vi "ElementPositions.vi"() -> ()   [LabVIEW 2012]
panel:
  in  "Threshold":dbl
  in  "ElementPositions":T1(array[cluster])
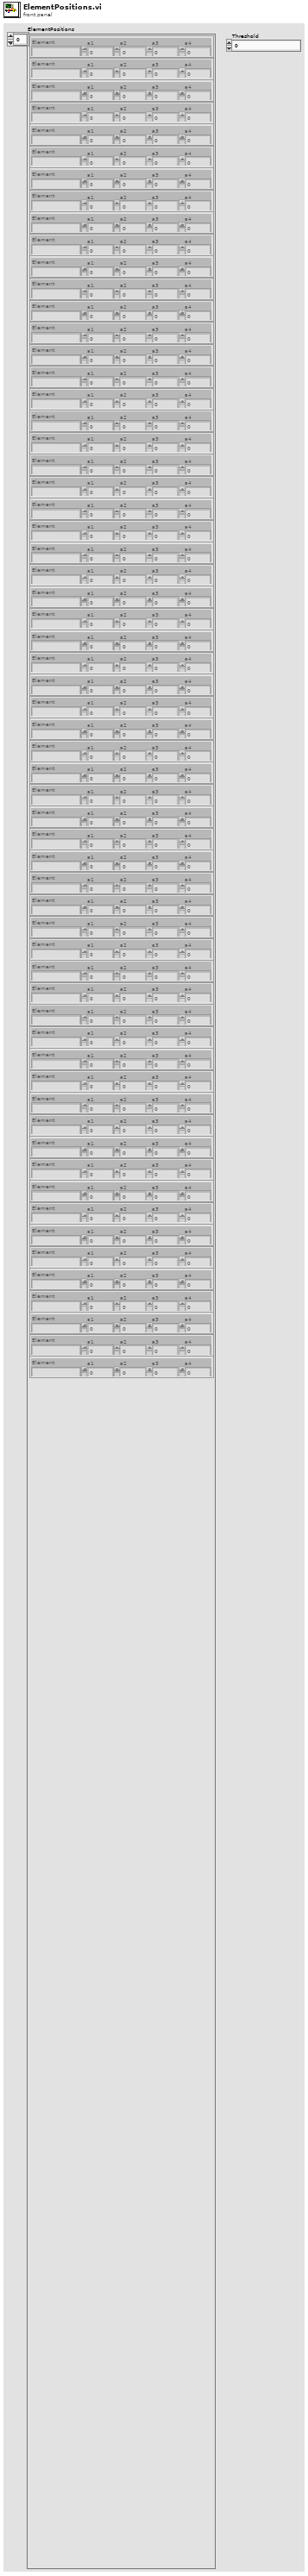
[diagram p1: front panel]
types:
  T1 = cluster{"Element":string, "a1":dbl, "a2":dbl, "a3":dbl, "a4":dbl}[]
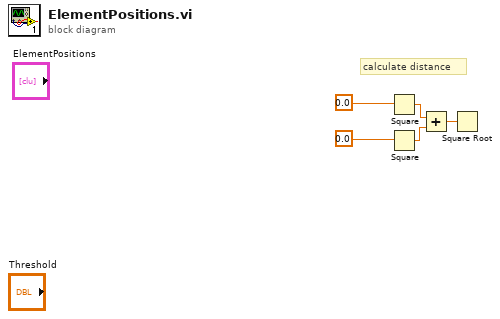
[diagram p0: block diagram]
diagram:
  # "calculate distance"
  n1 = Square(x=0.0) -> (x^2=w2:dbl)
  n2 = Square(x=0.0) -> (x^2=w3:dbl)
  n3 = Add(x=w2, y=w3) -> (x+y=w1:dbl)
  n4 = Square Root(x=w1) -> ()  [unwired: 1 out]
